vi "code validator.vi"(8 "error in":errorcluster, 9 "Card":refnum<vi>, 10 "User Input":string, 11 "Users indicate":T3) -> (0 "error out":errorcluster, 1 "Message":T1, 2 "Buttons":T2(ring), 3 "Users indicate":T3)   [LabVIEW 2015]
doc: "Validate user by checking code."
uses:
  controls/users ind.ctl
  controls/user.ctl
  controls/message.ctl
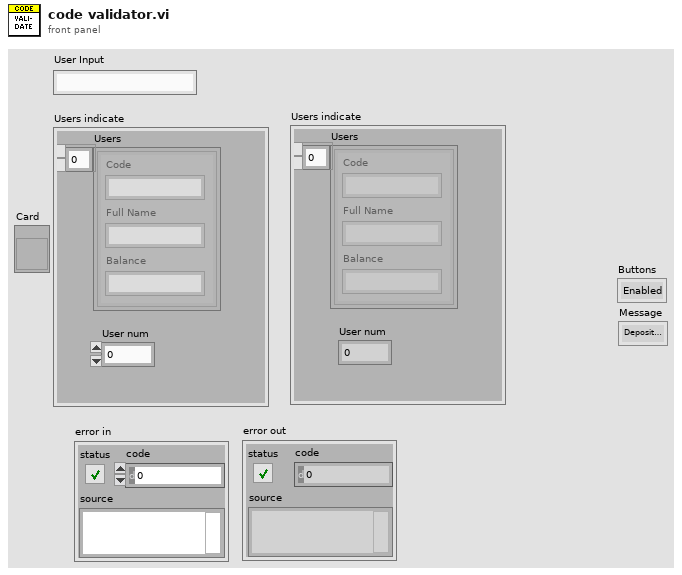
[diagram p1: front panel]
types:
  T1 = typedef "message.ctl" = enum16{"Deposit Complete", "Welcome", "Menu", "Verification Failed", "Session Terminate", "Deposit", "Withdrawal", "Withdrawal Complete", "Withdrawal Failed", "Balance Inq"}
  T2 = enum8{"Enabled", "Disabled", "Disabled and Grayed Out"}
  T3 = typedef "users ind.ctl" = cluster{"Users":T4[], "User num":i32}
  T4 = typedef "user.ctl" = cluster{"Code":string, "Full Name":string, "Balance":string}
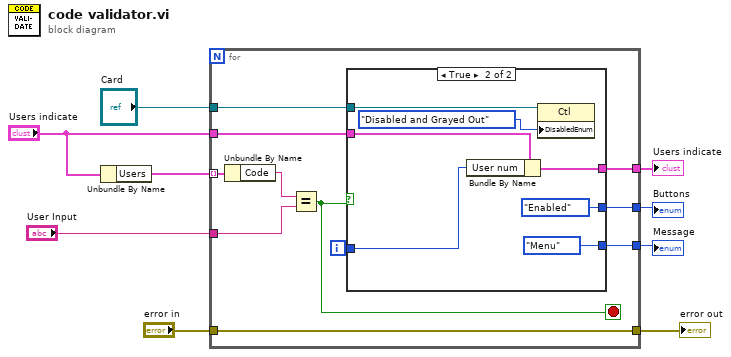
[diagram p0: block diagram]
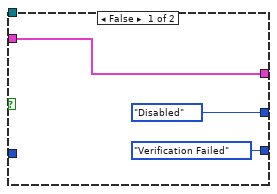
[diagram p2: hidden frame]
diagram:
  n1 = Unbundle By Name("Users indicate") -> ("Users"=w8:T4[])
  n2 = for {
    tunnel: "User Input" -> [w18]
    tunnel: w8 -> [w20] mode=indexing
    tunnel: [w17] -> w2
    tunnel: "Users indicate" -> [w15]
    tunnel: [w14] -> w4
    tunnel: [w13] -> w3
    tunnel: [w11] -> w6
    tunnel: "error in" -> [w11]
    tunnel: "Card" -> [w10]
    i -> [w16]
    stop <- w12 stop-if-true
    n3 = Unbundle By Name(w20) -> ("Code"=w19:string)
    n4 = Equal?(x=w19, y=w18) -> (x = y?=w12:bool)
    n5 = case shown="True" w12 {
      tunnel: [message."Verification Failed" ("Message in") message."Menu" ("Message in")] -> w17
      tunnel: w16 -> [_ w28]
      tunnel: w15 -> [w23 w29]
      tunnel: [w23 w27] -> w14
      tunnel: [T2."Disabled" ("Disabled") T2."Enabled" ("Disabled")] -> w13
      tunnel: w10 -> [_ w25]
      frame False {
      }
      frame True {
        n6 = Bundle By Name(cluster=w29, "User num"=w28) -> (w27:T3)
        n7 = property class="Ctl"(reference=w25, "DisabledEnum"=T2."Disabled and Grayed Out" ("Disabled")) -> ()  [unwired: 1 in, 2 out]
      }
    }
  }
  "error out" <- w6
  "Users indicate" <- w4
  "Buttons" <- w3
  "Message" <- w2
